vi "Host_main.vi"() -> ()   [LabVIEW 2013]
uses:
  <vilib>/userdefined/High Color/nirio_resource_hc.ctl
  FPGA/DataMode.ctl
  <vilib>/Analysis/4window.llb/windowTd.ctl
  Host/Scope/controls/power_spectrum_unit.ctl
  Host/Scope/P2P streaming/trigger_source.ctl
  Host/Scope/controls/Data_calc_mode.ctl
  Host/Scope/controls/Data_display_mode.ctl
  Host/Scope/controls/Graph_references.ctl
  Host/Scope/controls/graph_controls.ctl
  Host/Scope/controls/Channel_select.ctl
  Host/Scope/controls/ScopeMode.ctl
  <vilib>/FPGAPlugInAG/PXIe-7975R/niLvFpga_Open_PXIe-7975R.vi
  <vilib>/rvi/interface/common/dynamic/niFpgaDynamicAddResources.vi
  <vilib>/rvi/interface/common/niFpgaWaitOnOcc.vi
  <vilib>/Utility/error.llb/Error Cluster From Error Code.vi
  <vilib>/rvi/errors/niLvFpgaAdjustHostInterfaceError.vi
  <vilib>/FPGAPlugInAG/Dynamic/niLvFpga_Close_Dynamic.vi
  <vilib>/rvi/interface/nirviOpenFPGA/nirviOpenFPGA.xnode
  FPGA Bitfiles/mixer_FPGATarget2_FPGAmain_N0W7ub8HF6I.lvbitx
  <vilib>/rvi/interface/nirviReadWriteControl/nirviReadWriteControl.xnode
  Host/Config/FPGAref.ctl
  <vilib>/rvi/interface/nirviCloseFPGA/nirviCloseFPGA.xnode
  Host/Utilities/Ticker/Ticker.lvclass
  NiFpgaLv.dll
  <vilib>/rvi/interface/Simulation/niFpgaSimulationCallBeginRW.vi
  <vilib>/Analysis/NI_AALPro.lvlib
panel:
  out "error out":errorcluster
  in  "#bins":i32
  in  "ch1 DC offset":i16 caption="DC offset\nChannel 1"
  in  "ch0 DC offset":i16 caption="DC offset\nChannel 0"
  in  "Output delay delta":dbl(slide) scale=0.0..6.0
  in  "Output delay":dbl(slide) scale=0.0..6.0
  in  "Ch3":bool
  in  "Ch2":bool
  in  "Ch1":bool
  in  "Ch0":bool
  in  "Ch3 Q":bool
  in  "Ch3 I":bool
  in  "Ch2 Q":bool
  in  "Ch2 I":bool
  in  "input impedance":u32(ring) caption="Input Impedance" items=["1 mega ohm"=0, "50 ohms"=2]
  in  "SCOPE Resource":refnum<k15>="Dev1" caption="NI-Scope Resource"
  in  "Ch1 Q":bool
  in  "Ch1 I":bool
  in  "Ch0 Q":bool
  in  "Ch0 I":bool
  in  "Chart length":i32=400000
  in  "Refence for phase":T1
  in  "Graph_refs":T2
  out "Lower chart":dbl[][](graph)
  out "Upper chart":dbl[][](graph)
  out "Lower graph":i16[][](graph)
  in  "Buffer":T4
  in  "Display":T5
  in  "Output mixer fequency [MHz]":dbl
  in  "Trigger source":T6
  in  "Ch1 Q":bool
  in  "Ch1 I":bool
  in  "Ch0 Q":bool
  in  "Ch0 I":bool
  in  "Ch1":bool
  in  "Ch0":bool
  out "stop 2":bool
  in  "Zoom freq X":bool
  in  "Zoom freq Y":bool
  in  "Zoom time Y":bool
  in  "Zoom time X":bool
  in  "Unit":T7
  in  "Window":T8=1 items=["Rectangle"=0, "Hanning"=1, "Hamming"=2, "Blackman-Harris"=3, "Exact Blackman"=4, "Blackman"=5, "Flat Top"=6, "4 Term B-Harris "=7, "7 Term B-Harris"=8, "Low Sidelobe"=9, "Blackman Nuttall"=11, "Triangle"=30, "Bartlett-Hanning"=31, "Bohman"=32, "Parzen"=33, "Welch"=34, "Kaiser"=60, "Dolph-Chebyshev"=61, "Gaussian"=62]
  in  "Samples per 5782 record":i32
  in  "Phase offset (deg)":dbl
  in  "Fequency [MHz]":dbl
  in  "Mode":T9
  in  "Mixer freq [MHz]":dbl
  out "freqdata":cluster{"f0":dbl, "df":dbl, "magnitude":dbl[]}[](graph)
  out "Upper graph":i16[][](graph)
  in  "Rumode":bool
  in  "Singleshot":bool
  out "error IO":errorcluster
  in  "stop":bool
  in  "resource name":T10="RIO0"
  # "FPGA setup"
  # "ADU"
  # "ADU"
  # "Auto Zoom"
  # "Output delay"
  # "ns"
  # "Output delay delta"
  # "ps"
  # "Simulated data"
  # "5782"
  # "FFT"
  # "5160"
  # "Auto Zoom"
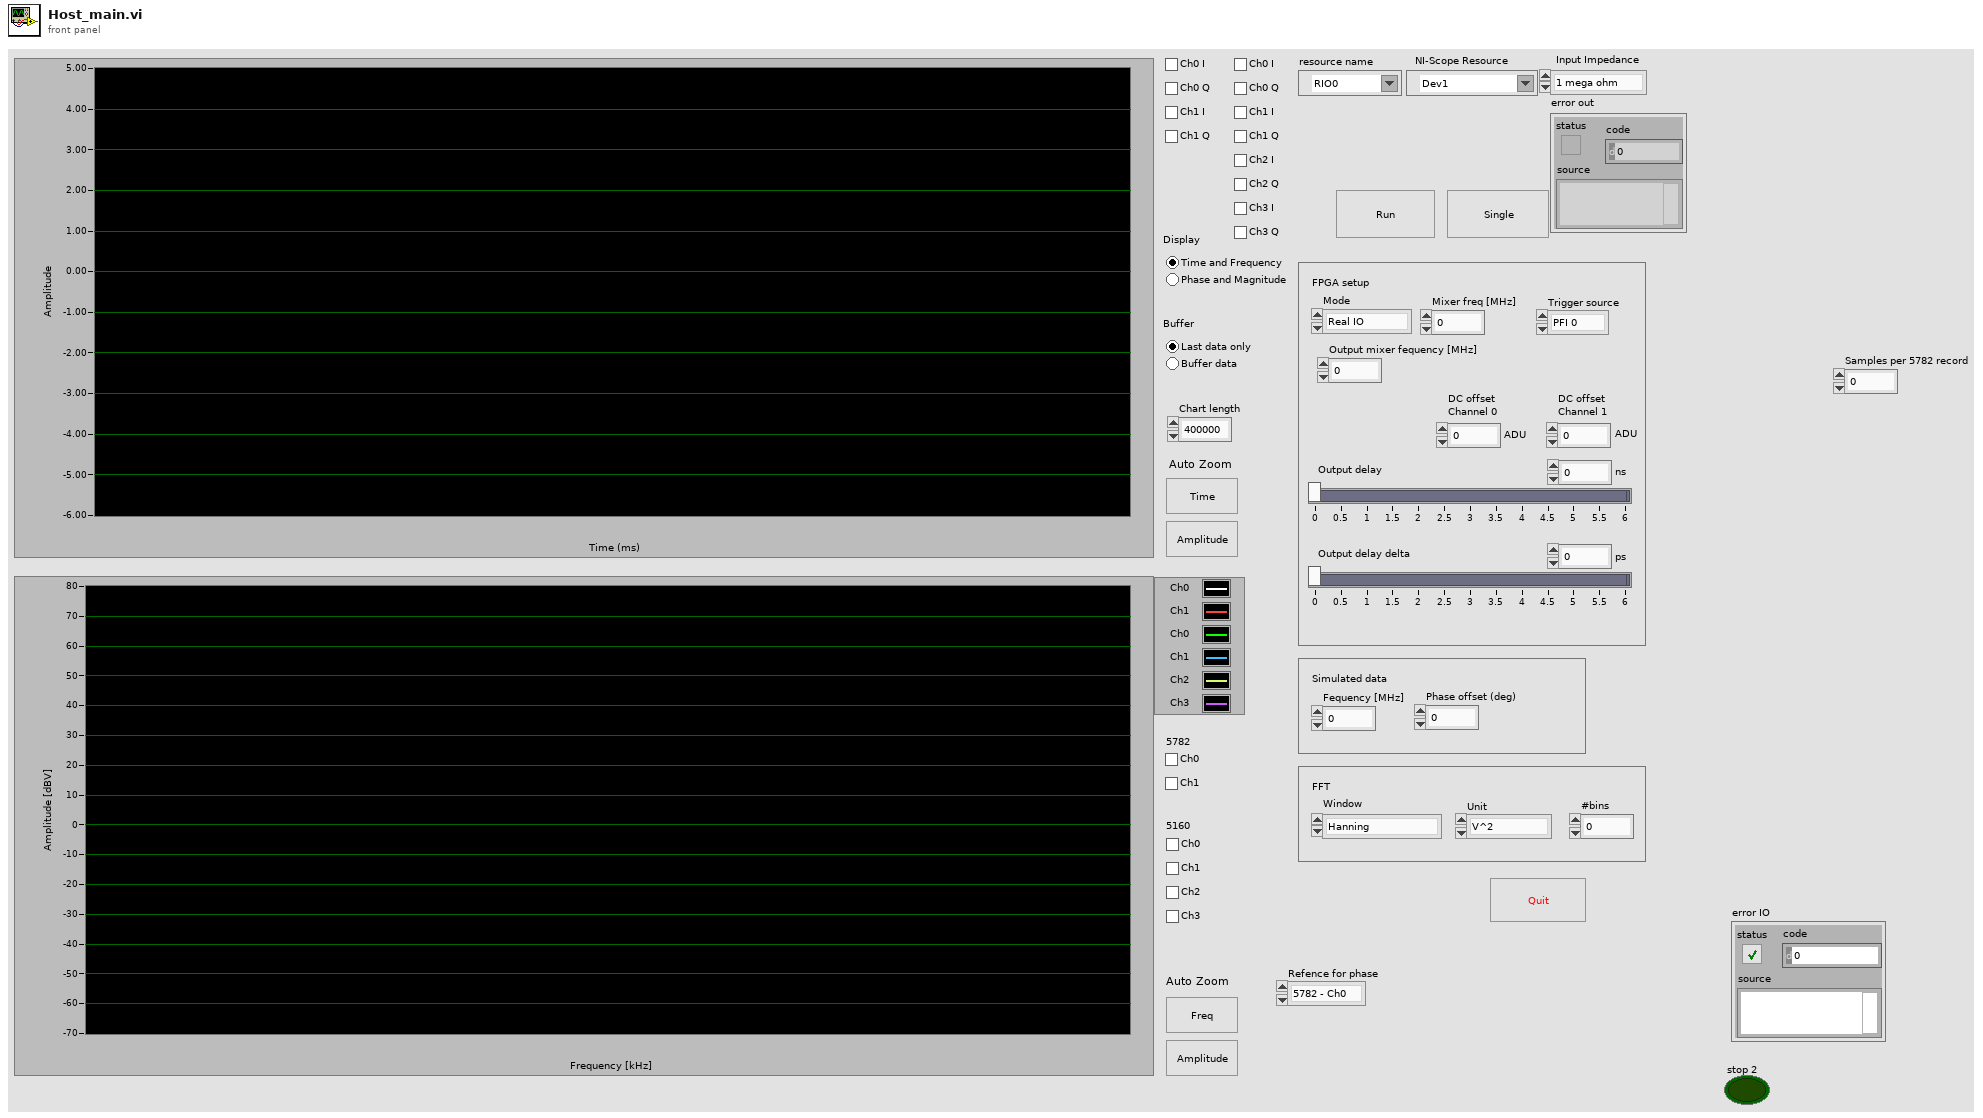
[diagram p1: front panel]
types:
  T1 = typedef "Channel_select.ctl" = enum16{"5782 - Ch0", "5782 - Ch1"}
  T2 = typedef "Graph_references.ctl" = cluster{"upper":T3, "lower":T3, "Freq graph":refnum<vi>}
  T3 = typedef "graph_controls.ctl" = cluster{"Graph":refnum<vi>, "Time btn":refnum<vi>, "Amplitude btn":refnum<vi>, "Chart":refnum<vi>}
  T4 = typedef "Data_display_mode.ctl" = enum32{"Last data only", "Buffer data"}
  T5 = typedef "Data_calc_mode.ctl" = enum32{"Time and Frequency", "Phase and Magnitude"}
  T6 = typedef "trigger_source.ctl" = enum16{"PFI 0", "PFI 1", "Software"}
  T7 = typedef "power_spectrum_unit.ctl" = enum16{"V^2", "V", "dBV"}
  T8 = typedef "NI_AALPro.lvlib/windowTd.ctl" = u32
  T9 = typedef "DataMode.ctl" = enum16{"Real IO", "Simulated"}
  T10 = typedef "nirio_resource_hc.ctl" = tag
  T11 = enum8{"Internal Clock PLL Off", "Internal Clock PLL On (REF IN)", "External Clock (CLK_IN)", "Internal Clock PLL On (IoModSyncClk)"}
  T12 = typedef "FPGAref.ctl" = refnum<k20>
  T13 = typedef "scope_params.ctl" = cluster{"scope mode":T14, "ticker":refnum<class "Ticker.lvclass">, "5160 samples per trigger":u32, "FPGA ref":T12, "P2P params":T15, "data mode":T9, "5782 samples per record":u32, "Chart length":i32}
  T14 = typedef "ScopeMode.ctl" = enum16{"Stopped", "Single", "Running", "Continuous"}
  T15 = typedef "P2P params.ctl" = cluster{"instrument handle":refnum<k15>, "stream session":refnum<k20>, "scale":cluster{"offset":dbl, "gain":dbl, "reserved 1":dbl, "reserved 2":dbl}, "actual sample rate":dbl, "Trigger":T6, "SCOPE Resource":refnum<k15>, "input impedance":u32}
  T16 = typedef "scope_params_5782.ctl" = cluster{"scope mode":T14, "ticker":refnum<class "Ticker.lvclass">, "samples per record":i32, "FPGA ref":T17, "data mode":T9, "5782 Trigger":T18, "Chart length":i32}
  T17 = typedef "FPGAref_5782.ctl" = refnum<k20>
  T18 = typedef "5782_trigger_type.ctl" = enum16{"Software", "Trigger input"}
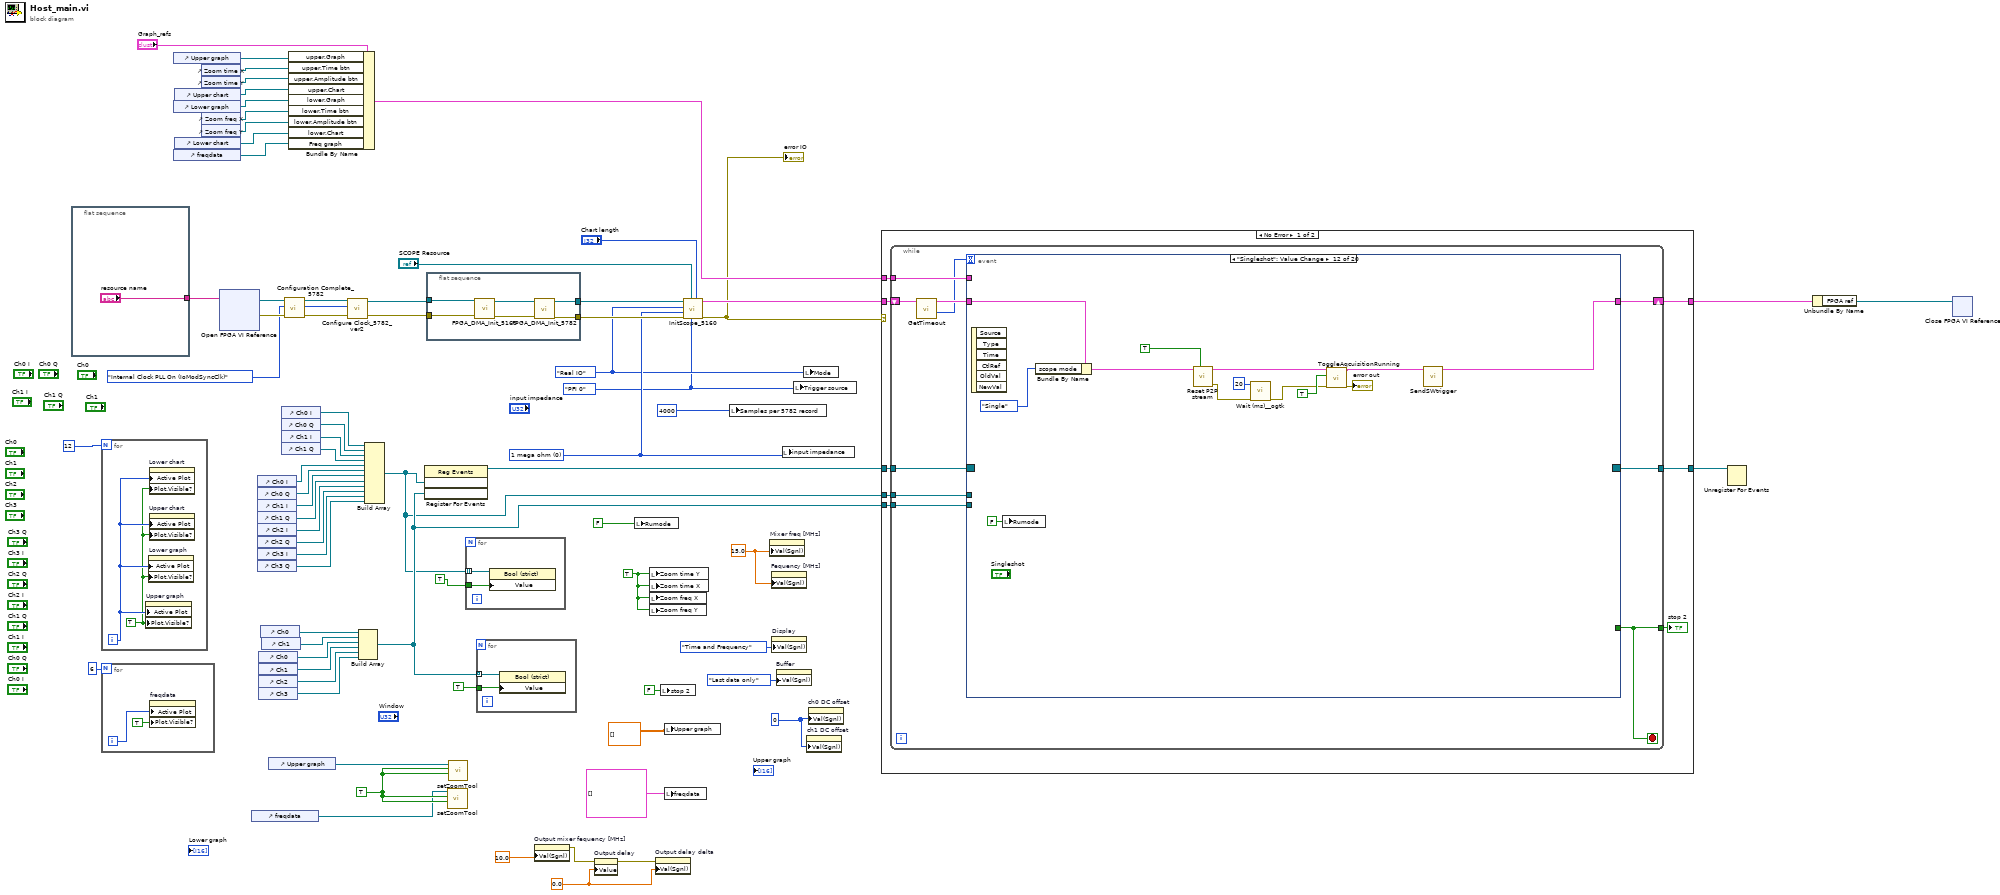
[diagram p0: block diagram]
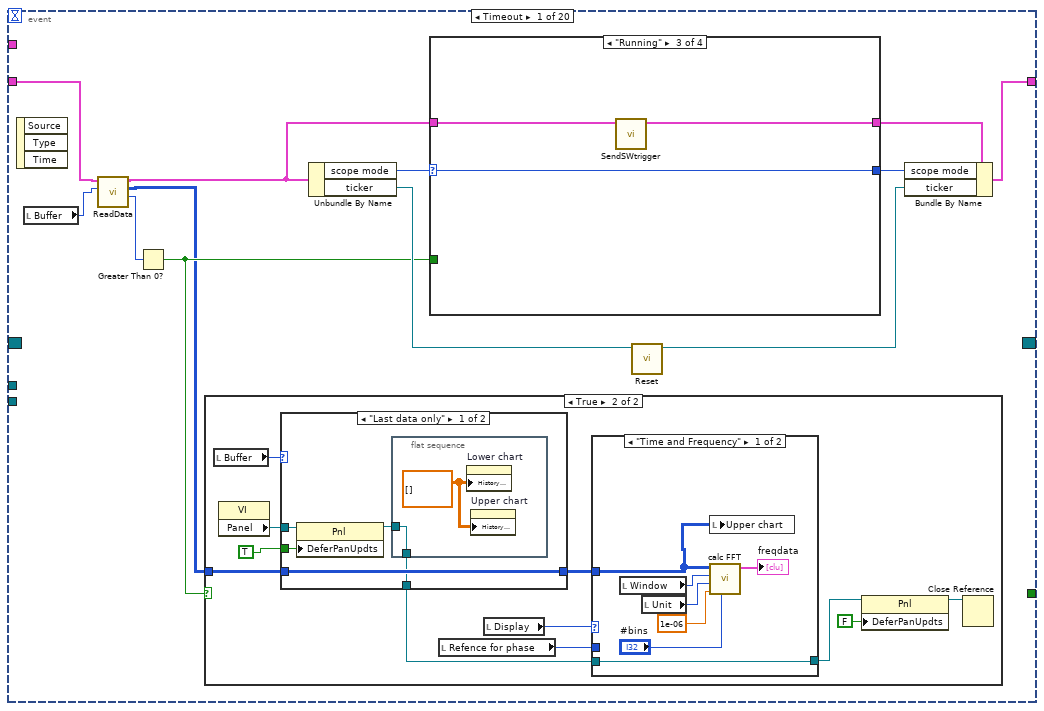
[diagram p2: hidden frame]
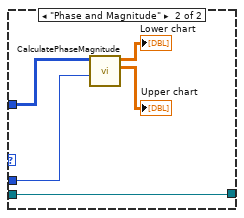
[diagram p5: hidden frame]
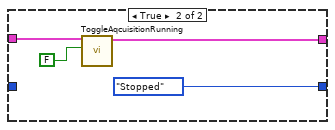
[diagram p9: hidden frame]
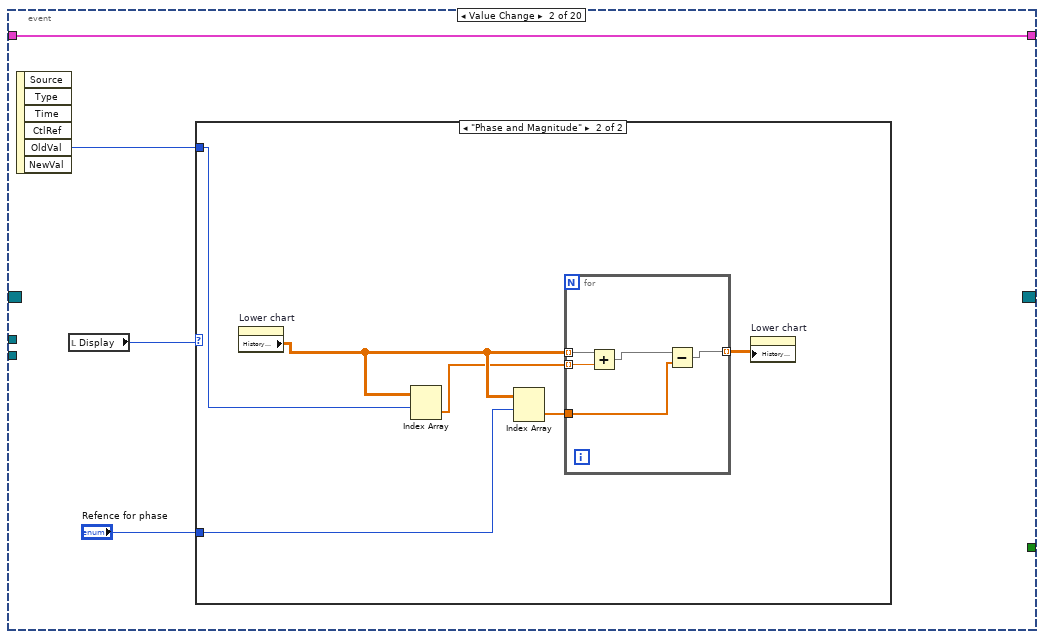
[diagram p10: hidden frame]
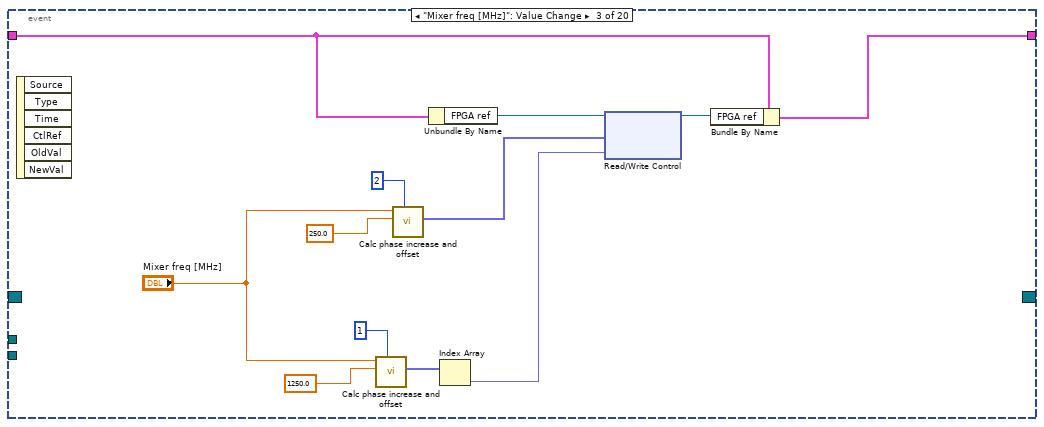
[diagram p12: hidden frame]
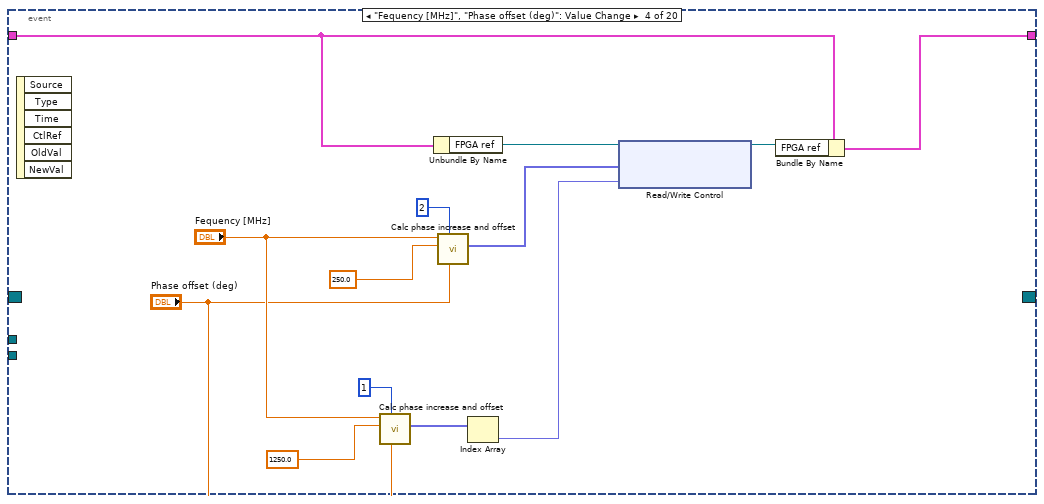
[diagram p13: hidden frame]
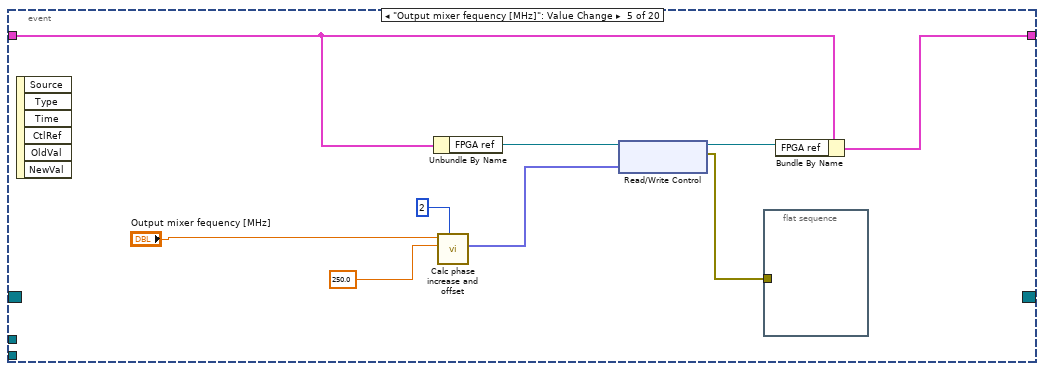
[diagram p14: hidden frame]
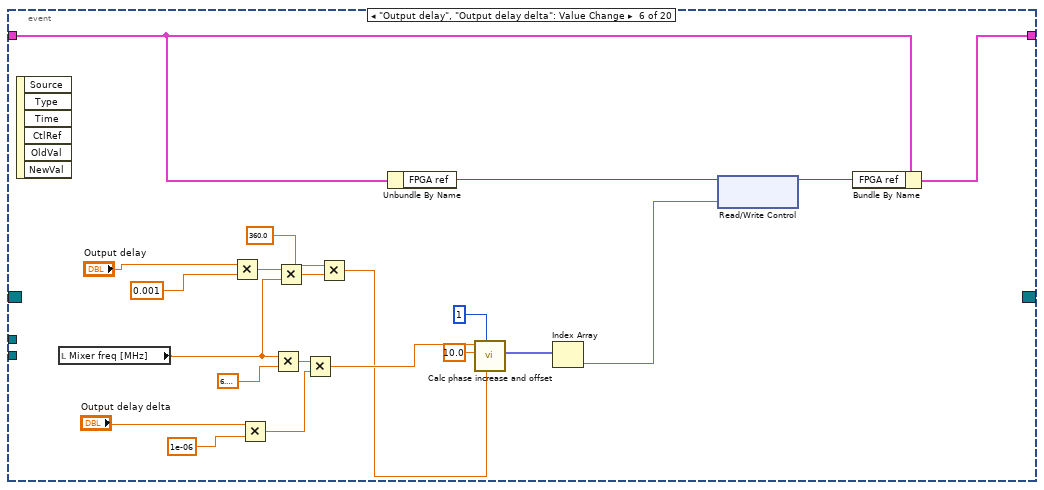
[diagram p15: hidden frame]
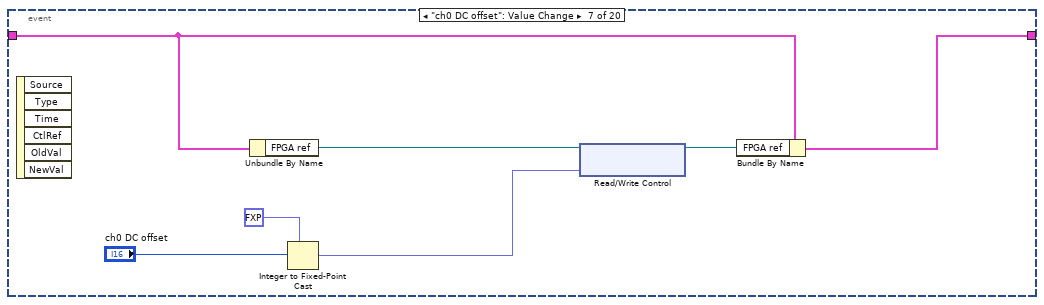
[diagram p16: hidden frame]
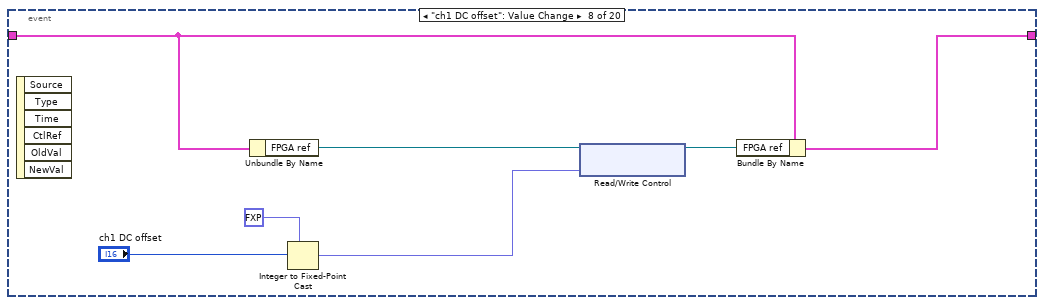
[diagram p17: hidden frame]
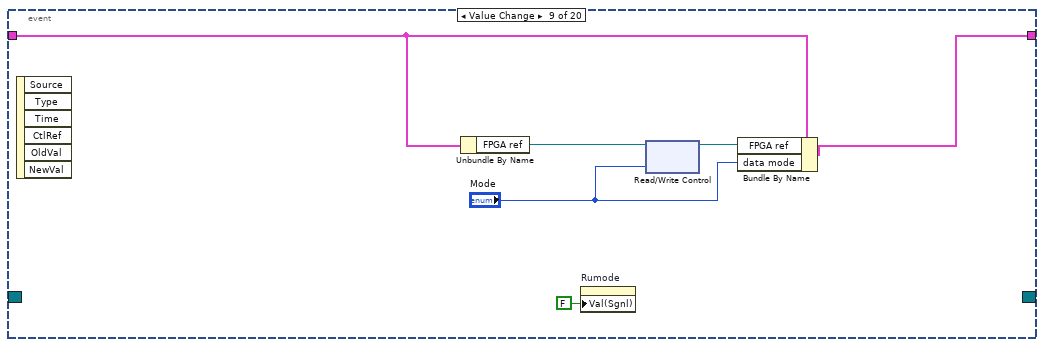
[diagram p18: hidden frame]
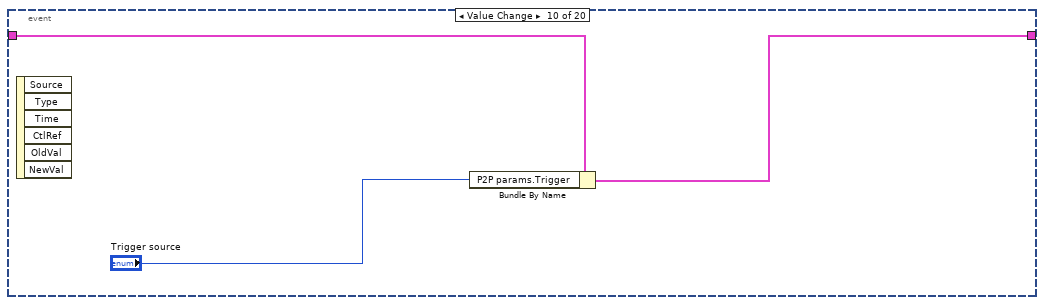
[diagram p19: hidden frame]
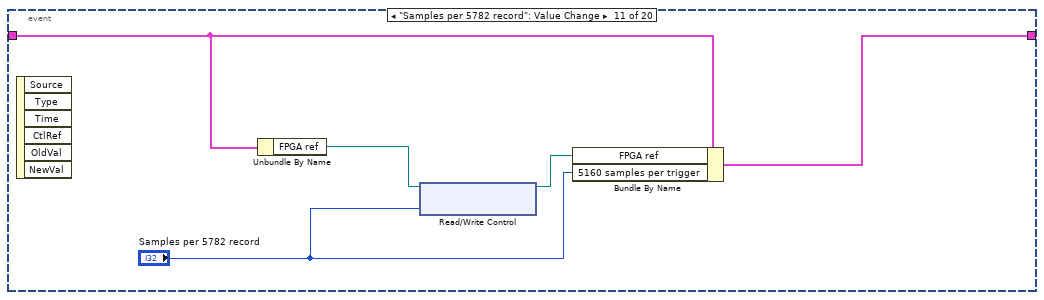
[diagram p20: hidden frame]
diagram:
  w5 = i16 0 ("Value (Signaling)")
  w9 = 0.0 ("Value (Signaling)")
  w13 = trigger_source."PFI 0" ("Trigger ource")
  w15 = u32 0 items=["1 mega ohm"=0, "50 ohms"=2] ("input impedance")
  w49 = TRUE ("Zoom  X")
  w58 = TRUE ("Rumode")
  w14 = DataMode."Real IO" ("Mode")
  w68 = 15.0 ("Mixer requency [MHz]")
  n1 = flat-sequence {
    tunnel: ["resource name"] -> w59
    frame #0 {
    }
  }
  n2 = for {
    N: 12 -> [_]
    i -> [w74]
    w73 = TRUE ("Plot.Visible")
    n3 = property on="Upper graph" class="WFGraph (strict)"("Active Plot"=w74, "Plot.Visible?"=w73) -> ()  [unwired: 2 in, 2 out]
    n4 = property on="Lower graph" class="WFGraph (strict)"("Active Plot"=w74, "Plot.Visible?"=w73) -> ()  [unwired: 2 in, 2 out]
    n5 = property on="Lower chart" class="WFChart (strict)"("Active Plot"=w74, "Plot.Visible?"=w73) -> ()  [unwired: 2 in, 2 out]
    n6 = property on="Upper chart" class="WFChart (strict)"("Active Plot"=w74, "Plot.Visible?"=w73) -> ()  [unwired: 2 in, 2 out]
  }
  n7 = for {
    N: 6 -> [_]
    i -> [w75]
    n8 = property on="freqdata" class="WFGraph (strict)"("Active Plot"=w75, "Plot.Visible?"=TRUE ("Plot.Visible")) -> ()  [unwired: 2 in, 2 out]
  }
  n9 = control-ref of="Upper graph"() -> (w43:refnum<vi>)
  n10 = control-ref of="Lower graph"() -> (w39:refnum<vi>)
  n11 = control-ref of="freqdata"() -> (w35:refnum<vi>)
  n12 = control-ref of="Upper chart"() -> (w40:refnum<vi>)
  n13 = control-ref of="Lower chart"() -> (w36:refnum<vi>)
  n14 = control-ref of="Zoom time X"() -> (w42:refnum<vi>)
  n15 = control-ref of="Zoom time Y"() -> (w41:refnum<vi>)
  n16 = control-ref of="Zoom freq X"() -> (w38:refnum<vi>)
  n17 = control-ref of="Zoom freq Y"() -> (w37:refnum<vi>)
  n18 = xnode "Open FPGA VI Reference"("resource name"=w59) -> ("FPGA VI Reference Out"=w4:refnum<k20>, "error out"=w19:errorcluster)  [unwired: 1 in]
  n19 = control-ref of="freqdata"() -> (w47:refnum<vi>)
  n20 = control-ref of="Ch0 I"() -> (w31:refnum<vi>)
  n21 = control-ref of="Ch0 Q"() -> (w30:refnum<vi>)
  n22 = control-ref of="Ch1 I"() -> (w29:refnum<vi>)
  n23 = control-ref of="Ch1 Q"() -> (w28:refnum<vi>)
  n24 = control-ref of="Ch2 I"() -> (w27:refnum<vi>)
  n25 = control-ref of="Ch2 Q"() -> (w26:refnum<vi>)
  n26 = control-ref of="Ch3 I"() -> (w25:refnum<vi>)
  n27 = control-ref of="Ch3 Q"() -> (w24:refnum<vi>)
  n28 = control-ref of="Ch0"() -> (w23:refnum<vi>)
  n29 = control-ref of="Ch1"() -> (w22:refnum<vi>)
  n30 = control-ref of="Ch2"() -> (w21:refnum<vi>)
  n31 = control-ref of="Ch3"() -> (w20:refnum<vi>)
  n32 = control-ref of="Ch0"() -> (w55:refnum<vi>)
  n33 = control-ref of="Ch1"() -> (w56:refnum<vi>)
  n34 = control-ref of="Upper graph"() -> (w48:refnum<vi>)
  n35 = control-ref of="Ch0 I"() -> (w51:refnum<vi>)
  n36 = control-ref of="Ch0 Q"() -> (w52:refnum<vi>)
  n37 = control-ref of="Ch1 I"() -> (w53:refnum<vi>)
  n38 = control-ref of="Ch1 Q"() -> (w54:refnum<vi>)
  n39 = call "Configuration Complete_5782.vi"("FPGA VI Reference in"=w4) -> ("FPGA VI Reference out"=w3:refnum<k20>)  [unwired: 8 in, 2 out]
  n40 = Bundle By Name(cluster="Graph_refs", "upper.Graph"=w43, "upper.Time btn"=w42, "upper.Amplitude btn"=w41, "upper.Chart"=w40, "lower.Graph"=w39, "lower.Time btn"=w38, "lower.Amplitude btn"=w37, "lower.Chart"=w36, "Freq graph"=w35) -> (w34:T2)
  n41 = call "Configure Clock_5782_ver2.vi"("Clock Source"=T11."Internal Clock PLL On (IoModSyncClk)", "FPGA VI Reference"=w3) -> ("FPGA VI Reference out"=w2:refnum<k20>)  [unwired: 7 in, 2 out]
  n42 = Build Array(w55, w56, w23, w22, w21, w20) -> (w60:refnum<vi>[])
  n43 = Build Array(w51, w52, w53, w54, w31, w30, w29, w28, w27, w26, w25, w24) -> (w50:refnum<vi>[])
  n44 = register-events(w50, w60) -> (reference out=w64:refnum<event-registration>)  [unwired: 2 in, 1 out]
  n45 = flat-sequence {
    tunnel: w19 -> [w82]
    tunnel: [w79] -> w18
    tunnel: w2 -> [w78]
    tunnel: [w77] -> w10
    frame #0 {
      n46 = call "FPGA_DMA_Init_5160.vi"("error in (no error)"=w82, "FPGA VI Reference"=w78) -> ("error out"=w80:errorcluster, "FPGA VI Reference out"=w81:T12)  [unwired: 7 in, 1 out]
      n47 = call "FPGA_DMA_Init_5782.vi"("error in (no error)"=w80, "FPGA VI Reference"=w81) -> ("error out"=w79:errorcluster, "FPGA VI Out"=w77:T12)  [unwired: 7 in, 1 out]
    }
  }
  n48 = call "setZoomTool.vi"("Zoom Y"=w49, "Zoom  X"=w49, "reference"=w47) -> ()  [unwired: 9 in]
  n49 = call "setZoomTool.vi"("Zoom Y"=w49, "Zoom  X"=w49, "reference"=w48) -> ()  [unwired: 9 in]
  n50 = for {
    tunnel: w50 -> [w84] mode=indexing
    tunnel: TRUE ("Rumode") -> [w83]
    n51 = property class="Bool (strict)"(reference=w84, "Value"=w83) -> ()  [unwired: 1 in, 2 out]
  }
  n52 = for {
    tunnel: w60 -> [w86] mode=indexing
    tunnel: TRUE ("Rumode") -> [w85]
    n53 = property class="Bool (strict)"(reference=w86, "Value"=w85) -> ()  [unwired: 1 in, 2 out]
  }
  n54 = property on="Output mixer fequency [MHz]" class="DigNum (strict)"("Val(Sgnl)"=10.0 ("Mixer requency [MHz]")) -> (error out=w8:errorcluster)  [unwired: 2 in, 1 out]
  n55 = property on="Output delay" class="Slide (strict)"(error in=w8, "Value"=w9) -> (error out=w7:errorcluster)  [unwired: 1 in, 1 out]
  n56 = local write "Rumode"(FALSE ("Rumode")) -> ()
  n57 = local write "Zoom time Y"(w58) -> ()
  n58 = local write "Zoom time X"(w58) -> ()
  n59 = local write "Zoom freq X"(w58) -> ()
  n60 = local write "Zoom freq Y"(w58) -> ()
  n61 = property on="Output delay delta" class="Slide (strict)"(error in=w7, "Val(Sgnl)"=w9) -> ()  [unwired: 1 in, 2 out]
  n62 = local write "stop 2"(FALSE ("stop 2")) -> ()
  n63 = local write "Upper graph"(dbl[][] [] ("Timedata")) -> ()
  n64 = local write "freqdata"(cluster{"f0":dbl, "df":dbl, "magnitude":dbl[]}[] [] ("freqdata")) -> ()
  n65 = call "InitScope_5160.vi"("Chart length"="Chart length", "Trigger ource"=w13, "SCOPE Resource"="SCOPE Resource", "error in"=w18, "input impedance"=w15, "data mode"=w14, "FPGA ref"=w10) -> ("error out"=w11:errorcluster, "scope params"=w12:T13)  [unwired: 3 in]
  "error IO" <- w11
  n66 = local write "Samples per 5782 record"(4000 ("Samples to aqcuire")) -> ()
  n67 = property on="Mixer freq [MHz]" class="DigNum (strict)"("Val(Sgnl)"=w68) -> ()  [unwired: 2 in, 2 out]
  n68 = property on="Fequency [MHz]" class="DigNum (strict)"("Val(Sgnl)"=w68) -> ()  [unwired: 2 in, 2 out]
  n69 = property on="Display" class="RadioBtnsControl (strict)"("Val(Sgnl)"=Data_calc_mode."Time and Frequency" ("Value (Signaling)")) -> ()  [unwired: 2 in, 2 out]
  n70 = property on="Buffer" class="RadioBtnsControl (strict)"("Val(Sgnl)"=enum32{"Last data only", "Buffer data"}."Last data only" ("Value (Signaling)")) -> ()  [unwired: 2 in, 2 out]
  n71 = local write "input impedance"(w15) -> ()
  n72 = local write "Trigger source"(w13) -> ()
  n73 = local write "Mode"(w14) -> ()
  n74 = property on="ch1 DC offset" class="DigNum (strict)"("Val(Sgnl)"=w5) -> ()  [unwired: 2 in, 2 out]
  n75 = property on="ch0 DC offset" class="DigNum (strict)"("Val(Sgnl)"=w5) -> ()  [unwired: 2 in, 2 out]
  n76 = case shown="No Error" w11 {
    tunnel: w12 -> [w94 w339]
    tunnel: [w93 w339] -> w45
    tunnel: w64 -> [w92 w338]
    tunnel: [w91 w338] -> w63
    tunnel: w50 -> [w90 _]
    tunnel: w60 -> [w89 _]
    tunnel: w34 -> [w87 _]
    frame No Error {
      n77 = while {
        shift-right: [w104] -> w93
        shift-left: w94 -> [w97]
        tunnel: w92 -> [w103]
        tunnel: [w102] -> w91
        tunnel: w90 -> [w101]
        tunnel: w89 -> [w100]
        tunnel: [w99] -> w88
        tunnel: w87 -> [w98]
        stop <- w99 stop-if-true
        n78 = call "GetTimeout.vi"("scope in"=w97) -> ("Time left"=w95:i32, "scope out"=w96:T13)  [unwired: 9 in]
        n79 = event shown="[11] \"Singleshot\": Value Change" {
          selector: w103 -> [_ _ _ _ _ _ _ _ _ _ _ _ _ _ _ _ _ _ _ _]
          dyn-events: [_ _ _ _ _ _ _ _ _ _ _ _ _ _ _ _ _ _ _ _] -> w102
          timeout: w95 -> [_ _ _ _ _ _ _ _ _ _ _ _ _ _ _ _ _ _ _ _]
          tunnel: [_ _ _ _ _ _ _ _ _ _ _ _ _ _ _ "stop" _ _ _ _] -> w99
          tunnel: w96 -> [w108 w170 w192 w202 w211 w221 w239 w246 w254 w258 w261 w275 w282 w303 w308 w309 w316 w324 w330 w337]
          tunnel: [w114 w170 w190 w201 w210 w219 w238 w245 w253 w257 w260 w269 w279 w303 w308 w309 w316 w324 w330 w337] -> w104
          tunnel: w101 -> [_ _ _ _ _ _ _ _ _ _ _ _ _ w302 _ _ _ _ _ _]
          tunnel: w100 -> [_ _ _ _ _ _ _ _ _ _ _ _ _ _ w306 _ _ _ _ _]
          tunnel: w98 -> [_ _ _ _ _ _ _ _ _ _ _ _ _ _ _ _ _ _ _ w334]
          event Timeout {
            n80 = event-data() -> ()  [unwired: 1 in, 3 out]
            n81 = local read "Buffer"() -> (w109:T4)
            n82 = call "ReadData.vi"("Buffer mode"=w109, "scope params"=w108) -> ("Num elements"=w106:i32, "data"=w107:i16[][], "scope params out"=w105:T13)  [unwired: 7 in]
            n83 = Greater Than 0?(x=w106) -> (x > 0?=w110:bool)
            n84 = case shown="True" w110 {
              tunnel: w107 -> [_ w124]
              frame False {
              }
              frame True {
                n85 = local read "Buffer"() -> (w126:T4)
                n86 = property class="VI"() -> ("Panel"=w119:refnum<vi>)  [unwired: 2 in, 2 out]
                n87 = case shown="\"Last data only\"" w126 {
                  tunnel: w124 -> [w132 w136]
                  tunnel: [w132 w136] -> w125
                  tunnel: w119 -> [w131 w135]
                  tunnel: TRUE ("Defer Panel Updates") -> [w129 _]
                  tunnel: [w128 w135] -> w117
                  frame "Last data only" {
                    n88 = property class="Pnl"(reference=w131, "DeferPanUpdts"=w129) -> (reference out=w130:refnum<vi>)  [unwired: 1 in, 1 out]
                    n89 = flat-sequence {
                      tunnel: w130 -> [w133]
                      tunnel: [w133] -> w128
                      frame #0 {
                        w134 = dbl[][] [] ("History Data")
                        n90 = property on="Lower chart" class="WFChart (strict)"("History Data"=w134) -> ()  [unwired: 2 in, 2 out]
                        n91 = property on="Upper chart" class="WFChart (strict)"("History Data"=w134) -> ()  [unwired: 2 in, 2 out]
                      }
                    }
                  }
                  frame "Buffer data" {
                  }
                }
                n92 = local read "Refence for phase"() -> (w123:T1)
                n93 = local read "Display"() -> (w127:T5)
                n94 = case shown="\"Time and Frequency\"" w127 {
                  tunnel: w125 -> [w139 w148]
                  tunnel: w123 -> [_ w145]
                  tunnel: [w138 w144] -> w121
                  tunnel: w117 -> [w138 w144]
                  frame "Time and Frequency" {
                    n95 = local read "Window"() -> (w140:T8)
                    n96 = local read "Unit"() -> (w141:T7)
                    n97 = local write "Upper chart"(w139) -> ()
                    n98 = call "calc FFT.vi"("#bins"="#bins", "dt"=1e-06, "Unit"=w141, "Window"=w140, "data"=w139) -> ("Power Spectrum / PSD"=→"freqdata":cluster{"f0":dbl, "df":dbl, "magnitude":dbl[]}[])  [unwired: 6 in]
                  }
                  frame "Phase and Magnitude" {
                    n99 = call "CalculatePhaseMagnitude.vi"("phase reference channel"=w145, "data"=w148) -> ("Magnitude"=→"Upper chart":dbl[][], "Phase"=→"Lower chart":dbl[][])  [unwired: 8 in]
                  }
                }
                n100 = property class="Pnl"(reference=w121, "DeferPanUpdts"=FALSE ("Defer Panel Updates")) -> (reference out=w120:refnum<vi>)  [unwired: 1 in, 1 out]
                n101 = Close Reference(reference=w120) -> ()  [unwired: 1 in, 1 out]
              }
            }
            n102 = Unbundle By Name(w105) -> ("scope mode"=w113:T14, "ticker"=w116:refnum<class "Ticker.lvclass">)
            n103 = case shown="\"Running\"" w113 {
              selector: w113 -> [w150 w152 w155 w156]
              tunnel: [w150 w152 w155 w160] -> w112
              tunnel: w105 -> [w149 w151 w154 w158]
              tunnel: [w149 w151 w153 w157] -> w111
              tunnel: w110 -> [_ _ _ w159]
              frame "Stopped" {
              }
              frame "Continuous" {
              }
              frame "Running" {
                n104 = call "SendSWtrigger.vi"("scope in"=w154) -> ("scope out"=w153:T13)  [unwired: 9 in, 1 out]
              }
              frame "Single" {
                n105 = case shown="False" w159 {
                  tunnel: [w161 ScopeMode."Stopped" ("scope mode")] -> w160
                  tunnel: w158 -> [w162 w165]
                  tunnel: [w162 w164] -> w157
                  tunnel: w156 -> [w161 _]
                  frame False {
                  }
                  frame True {
                    n106 = call "ToggleAqcuisitionRunning.vi"("Acquisition running"=FALSE, "scope in"=w165) -> ("scope out"=w164:T13)  [unwired: 8 in, 1 out]
                  }
                }
              }
            }
            n107 = call "Reset.vi"("Ticker in"=w116) -> ("Ticker out"=w115:refnum<class "Ticker.lvclass">)  [unwired: 9 in, 1 out]
            n108 = Bundle By Name(cluster=w111, "scope mode"=w112, "ticker"=w115) -> (w114:T13)
          }
          event Value Change {
            n109 = event-data() -> ("OldVal"=w167:T1)  [unwired: 1 in, 5 out]
            n110 = local read "Display"() -> (w168:T5)
            n111 = case shown="\"Phase and Magnitude\"" w168 {
              tunnel: "Refence for phase" -> [_ w175]
              tunnel: w167 -> [_ w173]
              frame "Time and Frequency", Default {
              }
              frame "Phase and Magnitude" {
                n112 = property on="Lower chart" class="WFChart (strict)"() -> ("History Data"=w174:dbl[][])  [unwired: 2 in, 2 out]
                n113 = Index Array(array=w174, index (row)=w173) -> (element=w172:dbl[])  [unwired: 1 in]
                n114 = Index Array(array=w174, index (row)=w175) -> (element=w176:dbl[])  [unwired: 1 in]
                n115 = for {
                  tunnel: w174 -> [w179] mode=indexing
                  tunnel: w176 -> [w181]
                  tunnel: [w180] -> w171 mode=indexing
                  tunnel: w172 -> [w178] mode=indexing
                  n116 = Add(x=w179, y=w178) -> (x+y=w177:dbl[])
                  n117 = Subtract(x=w177, y=w181) -> (x-y=w180:dbl[])
                }
                n118 = property on="Lower chart" class="WFChart (strict)"("History Data"=w171) -> ()  [unwired: 2 in, 2 out]
              }
            }
          }
          event "Mixer freq [MHz]": Value Change {
            n119 = event-data() -> ()  [unwired: 1 in, 6 out]
            n120 = call "Calc phase increase and offset.vi"("# of DDS"=1, "fclk (MHz)"=1250.0 ("fclk (800MHz)"), "f_generated (MHz)"="Mixer freq [MHz]") -> ("Phase out"=w184:fxp<+,64,64>[])  [unwired: 6 in, 2 out]
            n121 = call "Calc phase increase and offset.vi"("# of DDS"=2, "fclk (MHz)"=250.0 ("fclk (800MHz)"), "f_generated (MHz)"="Mixer freq [MHz]") -> ("Phase out"=w187:fxp<+,64,64>[])  [unwired: 6 in, 2 out]
            n122 = Unbundle By Name(w192) -> ("FPGA ref"=w193:T12)
            n123 = Index Array(array=w184) -> (element=w182:fxp<+,64,64>)  [unwired: 1 in]
            n124 = xnode "Read/Write Control"("FPGA VI Reference In"=w193, "Phase 5782"=w187, "phase 5160"=w182) -> ("FPGA VI Reference Out"=w191:T12)  [unwired: 1 in, 1 out]
            n125 = Bundle By Name(cluster=w192, "FPGA ref"=w191) -> (w190:T13)
          }
          event "Fequency [MHz]", "Phase offset (deg)": Value Change {
            n126 = event-data() -> ()  [unwired: 1 in, 6 out]
            n127 = call "Calc phase increase and offset.vi"("Phase offset (deg)"="Phase offset (deg)", "# of DDS"=1, "fclk (MHz)"=1250.0 ("fclk (800MHz)"), "f_generated (MHz)"="Fequency [MHz]") -> ("Phase out"=w197:fxp<+,64,64>[])  [unwired: 5 in, 2 out]
            n128 = Unbundle By Name(w202) -> ("FPGA ref"=w204:T12)
            n129 = call "Calc phase increase and offset.vi"("Phase offset (deg)"="Phase offset (deg)", "# of DDS"=2, "fclk (MHz)"=250.0 ("fclk (800MHz)"), "f_generated (MHz)"="Fequency [MHz]") -> ("Phase out"=w200:fxp<+,64,64>[])  [unwired: 5 in, 2 out]
            n130 = Index Array(array=w197) -> (element=w194:fxp<+,64,64>)  [unwired: 1 in]
            n131 = xnode "Read/Write Control"("FPGA VI Reference In"=w204, "Simulated phase 5782"=w200, "simulated phase 5160"=w194) -> ("FPGA VI Reference Out"=w203:T12)  [unwired: 1 in, 1 out]
            n132 = Bundle By Name(cluster=w202, "FPGA ref"=w203) -> (w201:T13)
          }
          event "Output mixer fequency [MHz]": Value Change {
            n133 = event-data() -> ()  [unwired: 1 in, 6 out]
            n134 = Unbundle By Name(w211) -> ("FPGA ref"=w213:T12)
            n135 = call "Calc phase increase and offset.vi"("# of DDS"=2, "fclk (MHz)"=250.0 ("fclk (800MHz)"), "f_generated (MHz)"="Output mixer fequency [MHz]") -> ("Phase out"=w209:fxp<+,64,64>[])  [unwired: 6 in, 2 out]
            n136 = xnode "Read/Write Control"("FPGA VI Reference In"=w213, "Phase output"=w209) -> ("FPGA VI Reference Out"=w212:T12, "error out"=w207:errorcluster)  [unwired: 1 in]
            n137 = flat-sequence {
              tunnel: w207 -> [_]
              frame #0 {
              }
            }
            n138 = Bundle By Name(cluster=w211, "FPGA ref"=w212) -> (w210:T13)
          }
          event "Output delay", "Output delay delta": Value Change {
            n139 = event-data() -> ()  [unwired: 1 in, 6 out]
            n140 = local read "Mixer freq [MHz]"() -> (w216:dbl)
            n141 = Multiply(x="Output delay", y=0.001) -> (x*y=w227:dbl)
            n142 = Multiply(x="Output delay delta", y=1e-06) -> (x*y=w228:dbl)
            n143 = Multiply(x=w216, y=6.283185307179586) -> (x*y=w233:dbl)
            n144 = Multiply(x=w227, y=w216) -> (x*y=w226:dbl)
            n145 = Multiply(x=w233, y=w228) -> (x*y=w232:dbl)
            n146 = Multiply(x=360.0, y=w226) -> (x*y=w224:dbl)
            n147 = Unbundle By Name(w221) -> ("FPGA ref"=w236:T12)
            n148 = call "Calc phase increase and offset.vi"("Phase offset (deg)"=w224, "# of DDS"=1, "fclk (MHz)"=10.0, "f_generated (MHz)"=w232) -> ("Phase out"=w223:fxp<+,64,64>[])  [unwired: 5 in, 2 out]
            n149 = Index Array(array=w223) -> (element=w222:fxp<+,64,64>)  [unwired: 1 in]
            n150 = xnode "Read/Write Control"("FPGA VI Reference In"=w236, "delay phase"=w222) -> ("FPGA VI Reference Out"=w220:T12)  [unwired: 1 in, 1 out]
            n151 = Bundle By Name(cluster=w221, "FPGA ref"=w220) -> (w219:T13)
          }
          event "ch0 DC offset": Value Change {
            n152 = event-data() -> ()  [unwired: 1 in, 6 out]
            n153 = Unbundle By Name(w239) -> ("FPGA ref"=w243:T12)
            n154 = Integer to Fixed-Point Cast(fixed-point type=fxp<+/-,16,16> 0.0 ("y"), integer="ch0 DC offset") -> (fixed-point=w240:fxp<+/-,16,16>)
            n155 = xnode "Read/Write Control"("FPGA VI Reference In"=w243, "DC offset chan 0"=w240) -> ("FPGA VI Reference Out"=w242:T12)  [unwired: 1 in, 1 out]
            n156 = Bundle By Name(cluster=w239, "FPGA ref"=w242) -> (w238:T13)
          }
          event "ch1 DC offset": Value Change {
            n157 = event-data() -> ()  [unwired: 1 in, 6 out]
            n158 = Unbundle By Name(w246) -> ("FPGA ref"=w250:T12)
            n159 = Integer to Fixed-Point Cast(fixed-point type=fxp<+/-,16,16> 0.0 ("y"), integer="ch1 DC offset") -> (fixed-point=w247:fxp<+/-,16,16>)
            n160 = xnode "Read/Write Control"("FPGA VI Reference In"=w250, "DC offset chan 0"=w247) -> ("FPGA VI Reference Out"=w249:T12)  [unwired: 1 in, 1 out]
            n161 = Bundle By Name(cluster=w246, "FPGA ref"=w249) -> (w245:T13)
          }
          event Value Change {
            n162 = event-data() -> ()  [unwired: 1 in, 6 out]
            n163 = Unbundle By Name(w254) -> ("FPGA ref"=w256:T12)
            n164 = property on="Rumode" class="Bool (strict)"("Val(Sgnl)"=FALSE ("Value (Signaling)")) -> ()  [unwired: 2 in, 2 out]
            n165 = xnode "Read/Write Control"("FPGA VI Reference In"=w256, "Mode"="Mode") -> ("FPGA VI Reference Out"=w255:T12)  [unwired: 1 in, 1 out]
            n166 = Bundle By Name(cluster=w254, "FPGA ref"=w255, "data mode"="Mode") -> (w253:T13)
          }
          event Value Change {
            n167 = event-data() -> ()  [unwired: 1 in, 6 out]
            n168 = Bundle By Name(cluster=w258, "P2P params.Trigger"="Trigger source") -> (w257:T13)
          }
          event "Samples per 5782 record": Value Change {
            n169 = event-data() -> ()  [unwired: 1 in, 6 out]
            n170 = Unbundle By Name(w261) -> ("FPGA ref"=w264:T12)
            n171 = xnode "Read/Write Control"("FPGA VI Reference In"=w264, "5782 record length"="Samples per 5782 record") -> ("FPGA VI Reference Out"=w263:T12)  [unwired: 1 in, 1 out]
            n172 = Bundle By Name(cluster=w261, "FPGA ref"=w263, "5160 samples per trigger"="Samples per 5782 record") -> (w260:T13)
          }
          event "Singleshot": Value Change {
            n173 = event-data() -> ()  [unwired: 1 in, 6 out]
            n174 = local write "Rumode"(FALSE ("Rumode")) -> ()
            n175 = Bundle By Name(cluster=w275, "scope mode"=ScopeMode."Single") -> (w273:T13)
            n176 = call "Reset P2P stream.vi"("single shot"=TRUE, "scope params"=w273) -> ("error out"=w267:errorcluster, "scope params out"=w271:T13)  [unwired: 8 in]
            n177 = call <userlib>:"Wait (ms)__ogtk.vi"("error in (no error)"=w267, "milliseconds to wait"=u32 20) -> ("error out"=w266:errorcluster)  [unwired: 8 in, 1 out]
            n178 = call "ToggleAqcuisitionRunning.vi"("error in"=w266, "Acquisition running"=TRUE, "scope in"=w271) -> ("error out"=→"error out":errorcluster, "scope out"=w270:T13)  [unwired: 7 in]
            n179 = call "SendSWtrigger.vi"("scope in"=w270) -> ("scope out"=w269:T13)  [unwired: 9 in, 1 out]
          }
          event "Rumode": Value Change {
            n180 = event-data() -> ()  [unwired: 1 in, 6 out]
            n181 = Select(t=ScopeMode."Running" ("scope mode"), s="Rumode", f=ScopeMode."Stopped" ("scope mode")) -> (s? t:f=w281:T14)
            n182 = Bundle By Name(cluster=w282, "scope mode"=w281) -> (w280:T13)
            n183 = case shown="\"Single\", \"Running\"" w281 {
              selector: w281 -> [w287 _ _]
              tunnel: w280 -> [w286 w292 w297]
              tunnel: [w285 w292 w296] -> w279
              frame "Single", "Running" {
                n184 = Equal?(x=ScopeMode."Single" ("scope mode"), y=w287) -> (x = y?=w288:bool)
                n185 = call "Reset P2P stream.vi"("single shot"=w288, "scope params"=w286) -> ("scope params out"=w291:T13)  [unwired: 8 in, 1 out]
                n186 = call "ToggleAqcuisitionRunning.vi"("Acquisition running"=TRUE, "scope in"=w291) -> ("scope out"=w285:T13)  [unwired: 8 in, 1 out]
              }
              frame "Continuous" {
                n187 = disable-structure shown="Disabled" {
                  frame Disabled {
                    n188 = call "ToggleAqcuisitionRunning_5782.vi"("Acquisition running"=TRUE) -> ("scope out"=w294:T16)  [unwired: 9 in, 1 out]
                    n189 = call "ToggleContinousMode.vi"("Cont Acquisition"=TRUE ("Acquisition running"), "scope in"=w294) -> ()  [unwired: 8 in, 2 out]
                  }
                  frame Enabled {
                  }
                }
              }
              frame "Stopped" {
                n190 = call "ToggleAqcuisitionRunning.vi"("Acquisition running"=FALSE, "scope in"=w297) -> ("scope out"=w296:T13)  [unwired: 8 in, 1 out]
              }
            }
          }
          event Value Change {
            n191 = event-data() -> ("CtlRef"=w301:refnum<vi>, "NewVal"=w299:bool)  [unwired: 1 in, 4 out]
            n192 = Search 1D Array(1D array=w302, element=w301) -> (index of element=w300:i32)  [unwired: 1 in]
            n193 = property on="Upper graph" class="WFGraph (strict)"("Active Plot"=w300, "Plot.Visible?"=w299) -> ()  [unwired: 2 in, 2 out]
            n194 = property on="Upper chart" class="WFChart (strict)"("Active Plot"=w300, "Plot.Visible?"=w299) -> ()  [unwired: 2 in, 2 out]
          }
          event Value Change {
            n195 = event-data() -> ("CtlRef"=w307:refnum<vi>, "NewVal"=w304:bool)  [unwired: 1 in, 4 out]
            n196 = Search 1D Array(1D array=w306, element=w307) -> (index of element=w305:i32)  [unwired: 1 in]
            n197 = property on="freqdata" class="WFGraph (strict)"("Active Plot"=w305, "Plot.Visible?"=w304) -> ()  [unwired: 2 in, 2 out]
            n198 = property on="Lower chart" class="WFChart (strict)"("Active Plot"=w305, "Plot.Visible?"=w304) -> ()  [unwired: 2 in, 2 out]
          }
          event "stop": Value Change {
            n199 = event-data() -> ()  [unwired: 1 in, 6 out]
          }
          event Value Change {
            n200 = event-data() -> ()  [unwired: 1 in, 6 out]
            n201 = case shown="\"V\"" "Unit" {
              tunnel: ["V" "dBV" "V^2"] -> w313
              frame "V" {
              }
              frame "dBV" {
              }
              frame "V^2" {
              }
            }
            n202 = Concatenate Strings("Amplitude [", w313, "]") -> (w311:string)
            n203 = property on="freqdata" class="WFGraph (strict)"("YScale.NameLbl.Text"=w311) -> ()  [unwired: 2 in, 2 out]
          }
          event "Zoom time X", "Zoom time Y": Value Change {
            n204 = event-data() -> ()  [unwired: 1 in, 6 out]
            n205 = control-ref of="Upper chart"() -> (w322:refnum<vi>)
            n206 = control-ref of="Upper graph"() -> (w323:refnum<vi>)
            n207 = call "setZoomTool.vi"("Zoom Y"="Zoom time Y", "Zoom  X"="Zoom time X", "reference"=w322) -> ()  [unwired: 9 in]
            n208 = call "setZoomTool.vi"("Zoom Y"="Zoom time Y", "Zoom  X"="Zoom time X", "reference"=w323) -> ()  [unwired: 9 in]
          }
          event "Zoom freq Y", "Zoom freq X": Value Change {
            n209 = event-data() -> ()  [unwired: 1 in, 6 out]
            n210 = control-ref of="Lower chart"() -> (w328:refnum<vi>)
            n211 = control-ref of="Lower graph"() -> (w327:refnum<vi>)
            n212 = control-ref of="freqdata"() -> (w329:refnum<vi>)
            n213 = call "setZoomTool.vi"("Zoom Y"="Zoom freq Y", "Zoom  X"="Zoom freq X", "reference"=w329) -> ()  [unwired: 9 in]
            n214 = call "setZoomTool.vi"("Zoom Y"="Zoom freq Y", "Zoom  X"="Zoom freq X", "reference"=w328) -> ()  [unwired: 9 in]
            n215 = call "setZoomTool.vi"("Zoom Y"="Zoom freq Y", "Zoom  X"="Zoom freq X", "reference"=w327) -> ()  [unwired: 9 in]
          }
          event Value Change {
            w333 = dbl[][] [] ("History Data")
            n216 = event-data() -> ()  [unwired: 1 in, 6 out]
            n217 = property on="Upper chart" class="WFChart (strict)"("History Data"=w333) -> ()  [unwired: 2 in, 2 out]
            n218 = property on="Lower chart" class="WFChart (strict)"("History Data"=w333) -> ()  [unwired: 2 in, 2 out]
            n219 = local write "freqdata"(cluster{"f0":dbl, "df":dbl, "magnitude":dbl[]}[] [] ("freqdata")) -> ()
            n220 = call "UpdateGraphs.vi"("Buffer mode"="Buffer", "Display mode"="Display", "Graph_refs"=w334) -> ()  [unwired: 9 in]
            n221 = property on="Zoom time X" class="Bool (strict)"("Val(Sgnl)"=TRUE ("Value (Signaling)")) -> ()  [unwired: 2 in, 2 out]
          }
        }
      }
      "stop 2" <- w88
    }
    frame Error {
    }
  }
  n222 = Unregister For Events(event registration refnum=w63) -> ()  [unwired: 1 in, 1 out]
  n223 = Unbundle By Name(w45) -> ("FPGA ref"=w71:T12)
  n224 = xnode "Close FPGA VI Reference"("FPGA VI Reference In"=w71) -> ()  [unwired: 1 in, 1 out]
